vi "DAQ_DC Voltage Gen Configure and Generate.vi"(0 "DAQmx Task In":refnum<k21>, 5 "Output Voltages (V)":dbl[](array[numeric]) format="%.2p", 7 "Range Settings":T1={"Min Range(V)"=-10.0, "Max Range(V)"=10.0} {"Max Range(V)" format="%.2p"; "Min Range(V)" format="%.2p"}, 11 "error in":errorcluster) -> (4 "DAQmx Task Out":refnum<k21>, 15 "error out":errorcluster)   [LabVIEW 2021, in "DAQ_DC Voltage Generation.lvlib"]
doc: "Configure and generate DC Voltage on the channels configured."
uses:
  DAQ_DC Voltage Generation.lvlib
  Typedefs/Range Settings.ctl
  <vilib>/DAQmx/write.llb/DAQmx Write (Analog 1D DBL NChan 1Samp).vi
  <vilib>/DAQmx/miscellaneous.llb/DAQmx Fill In Error Info.vi
  <resource>/objmgr/daqmx.rc
panel:
  # "Inputs"
  # "Range Settings"
  # "Output Settings"
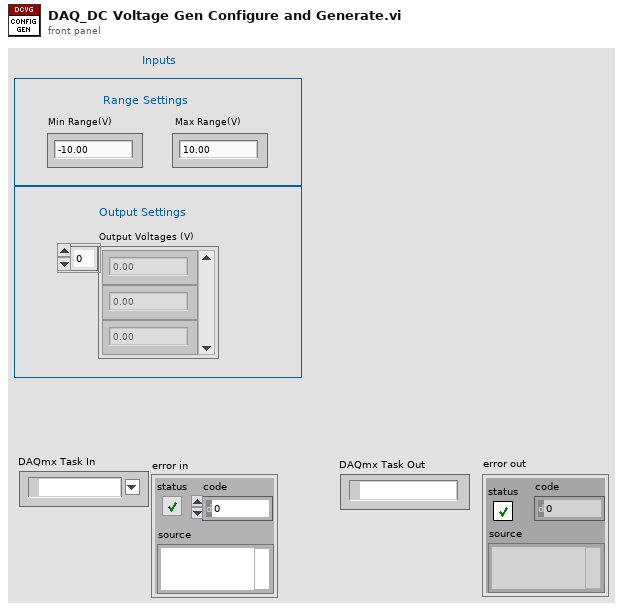
[diagram p1: front panel]
types:
  T1 = typedef "DAQ_DC Voltage Generation.lvlib/Range Settings.ctl" = cluster{"Min Range(V)":dbl, "Max Range(V)":dbl}
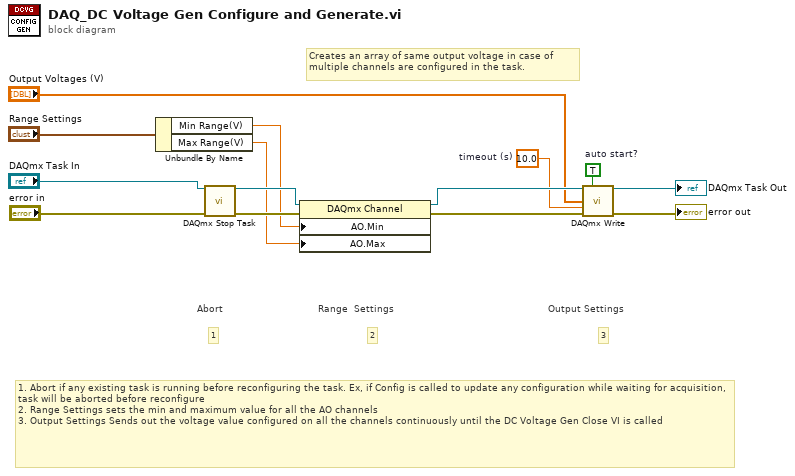
[diagram p0: block diagram]
diagram:
  w1 = 10.0  # timeout (s)
  w9 = TRUE  # auto start?
  # "1"
  # "Abort"
  # "Creates an array of same output voltage in case of multiple channels are configured in the task."
  # "3"
  # "Output Settings"
  # "2"
  # "Range  Settings"
  # "1. Abort if any existing task is running before reconfiguring the task. Ex, if Config is called to update any configuration while waiting for acquisition, task will be aborted before reconfigure\n2. Range Settings sets the min and maximum value for all the AO channels\n3. Output Settings Sends out the voltage value configured on all the channels continuously until the DC Voltage Gen Close VI is called"
  n1 = Unbundle By Name("Range Settings") -> ("Min Range(V)"=w4:dbl, "Max Range(V)"=w3:dbl)
  n2 = call <vilib>:"DAQmx Stop Task.vi"("task/channels in"="DAQmx Task In", "error in"="error in") -> ("task out"=w10:refnum<k21>, "error out"=w6:errorcluster)  [unwired: 12 in]
  n3 = property class="DAQmx Channel"(reference=w10, error in=w6, "AO.Min"=w4, "AO.Max"=w3) -> (reference out=w11:refnum<k21>, error out=w12:errorcluster)
  n4 = call-poly <vilib>:"DAQmx Write.vi"("task/channels in"=w11, "auto start"=w9, "data"="Output Voltages (V)", "timeout"=w1, "error in"=w12) -> ("task out"=→"DAQmx Task Out":refnum<k21>, "error out"=→"error out":errorcluster)  [unwired: 8 in, 1 out]
